vi "Kaelus PFE Config Test.vi"(8 "error in (no error)":errorcluster, 10 "Configuration":T2={"BusType"=enum."USB", "Card"=0, "USB"="", "IP"=0, "COM"=1, "Baud Rate"=enum."9600"}, 11 "Str Refnum":refnum<vi>) -> (0 "error out":errorcluster, 3 "Kaelus PFE":T1)   [LabVIEW 2011]
uses:
  TypeDefs/Kaelus PFE Configuration.ctl
  TypeDefs/Kaelus PFE Instrument Info.ctl
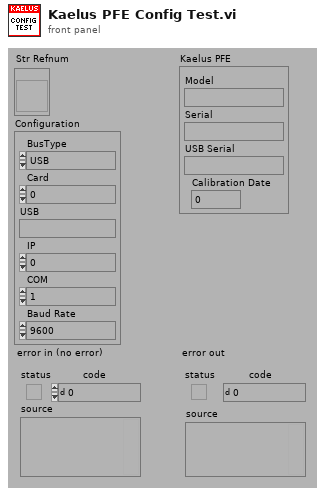
[diagram p1: front panel]
types:
  T1 = typedef "Kaelus PFE Instrument Info.ctl" = cluster{"Model":string, "Serial":string, "USB Serial":string, "Calibration Date":dbl}
  T2 = typedef "Kaelus PFE Configuration.ctl" = cluster{"BusType":enum32{"PCI/ISA/PCMCIA", "USB", "Ethernet", "Serial"}, "Card":i32, "USB":string, "IP":u32, "COM":i32, "Baud Rate":enum16{"300", "600", "1200", "2400", "4800", "9600"}}
  T3 = enum32{"PCI/ISA/PCMCIA", "USB", "Ethernet", "Serial"}
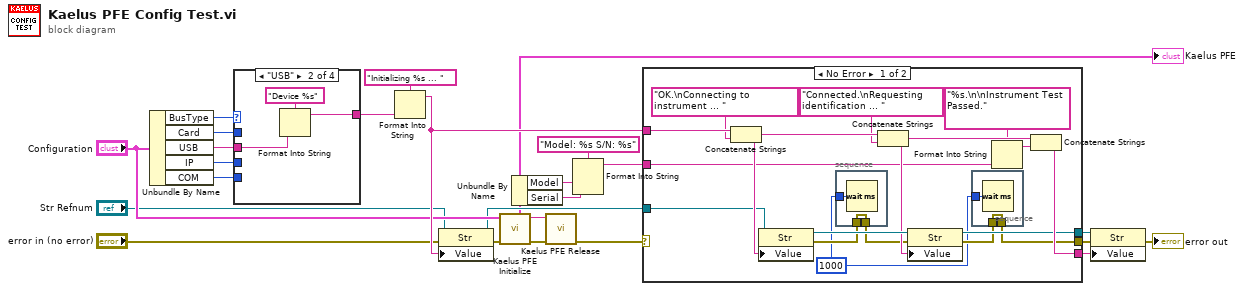
[diagram p0: block diagram]
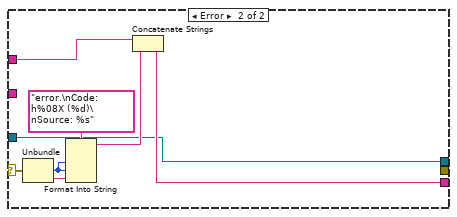
[diagram p2: hidden frame]
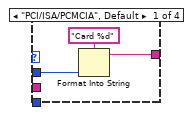
[diagram p3: hidden frame]
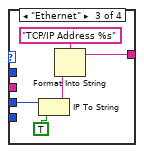
[diagram p4: hidden frame]
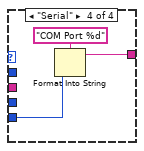
[diagram p5: hidden frame]
diagram:
  n1 = Unbundle By Name("Configuration") -> ("BusType"=w24:T3, "Card"=w23:i32, "USB"=w22:string, "IP"=w21:u32, "COM"=w20:i32)
  n2 = case shown="\"USB\"" w24 {
    tunnel: w23 -> [w27 _ _ _]
    tunnel: w22 -> [_ w29 _ _]
    tunnel: w21 -> [_ _ w35 _]
    tunnel: w20 -> [_ _ _ w37]
    tunnel: [w26 w30 w32 w38] -> w19
    frame "PCI/ISA/PCMCIA", Default {
      n3 = Format Into String(format string="Card %d", w27) -> (resulting string=w26:string)  [unwired: 2 in, 1 out]
    }
    frame "USB" {
      n4 = Format Into String(format string="Device %s", w29) -> (resulting string=w30:string)  [unwired: 2 in, 1 out]
    }
    frame "Ethernet" {
      n5 = IP To String(1:TRUE, 2:w35) -> (0:w34:string)
      n6 = Format Into String(format string="TCP/IP Address %s", w34) -> (resulting string=w32:string)  [unwired: 2 in, 1 out]
    }
    frame "Serial" {
      n7 = Format Into String(format string="COM Port %d", w37) -> (resulting string=w38:string)  [unwired: 2 in, 1 out]
    }
  }
  n8 = Format Into String(format string="Initializing %s ... ", w19) -> (resulting string=w18:string)  [unwired: 2 in, 1 out]
  n9 = property class="Str"(reference="Str Refnum", error in="error in (no error)", "Value"=w18) -> (reference out=w4:refnum<vi>, error out=w16:errorcluster)
  n10 = call "Kaelus PFE Initialize.vi"("error in (no error)"=w16, "Configuration"="Configuration") -> ("error out"=w14:errorcluster, "DAQmx Dev Name (FEModule)"=w12:string, "Kaelus PFE"=w1:T1)  [unwired: 7 out]
  "Kaelus PFE" <- w1
  n11 = Unbundle By Name(w1) -> ("Model"=w3:string, "Serial"=w2:string)
  n12 = call "Kaelus PFE Release.vi"("error in (no error)"=w14, "DAQmx Dev Name (FEModule)"=w12) -> ("error out"=w13:errorcluster)  [unwired: 1 in, 8 out]
  n13 = Format Into String(format string="Model: %s S/N: %s" ("Return Model and Serial #"), w3, w2) -> (resulting string=w11:string)  [unwired: 2 in, 1 out]
  n14 = case shown="No Error" w13 {
    selector: w13 -> [_ w66]
    tunnel: w18 -> [w55 w68]
    tunnel: w4 -> [w50 w61]
    tunnel: w11 -> [w47 _]
    tunnel: [w46 w62] -> w9
    tunnel: [w45 w61] -> w7
    tunnel: [w41 _] -> w6
    frame No Error {
      w40 = u32 1000 ("milliseconds to wait")
      n15 = Concatenate Strings(w55, "OK.\nConnecting to instrument ... ") -> (w53:string)
      n16 = property class="Str"(reference=w50, "Value"=w53) -> (reference out=w56:refnum<vi>, error out=w44:errorcluster)  [unwired: 1 in]
      n17 = stacked-sequence {
        tunnel: w40 -> [w60]
        tunnel: w44 -> [w59]
        tunnel: [w59] -> w43
        frame #0 {
          n18 = Wait (ms)(milliseconds to wait=w60) -> ()  [unwired: 1 out]
        }
      }
      n19 = Concatenate Strings(w53, "Connected.\nRequesting identification ... ") -> (w51:string)
      n20 = property class="Str"(reference=w56, error in=w43, "Value"=w51) -> (reference out=w45:refnum<vi>, error out=w42:errorcluster)
      n21 = stacked-sequence {
        tunnel: w40 -> [w58]
        tunnel: w42 -> [w57]
        tunnel: [w57] -> w41
        frame #0 {
          n22 = Wait (ms)(milliseconds to wait=w58) -> ()  [unwired: 1 out]
        }
      }
      n23 = Format Into String(format string="%s.\n\nInstrument Test Passed.", w47) -> (resulting string=w48:string)  [unwired: 2 in, 1 out]
      n24 = Concatenate Strings(w51, w48) -> (w46:string)
    }
    frame Error {
      n25 = Unbundle(w66) -> ("code"=w65:i32, "source"=w64:string)  [unwired: 1 out]
      n26 = Format Into String(format string="error.\nCode:  h%08X (%d)\nSource: %s", w65, w65, w64) -> (resulting string=w63:string)  [unwired: 2 in, 1 out]
      n27 = Concatenate Strings(w68, w63) -> (w62:string)
    }
  }
  n28 = property class="Str"(reference=w7, error in=w6, "Value"=w9) -> (error out=→"error out":errorcluster)  [unwired: 1 out]
